vi "bah.vi"() -> ()   [LabVIEW 2013]
panel:
  in  "OK Button 2":bool
  in  "Один раз(T)/50 раз (F)":bool
  in  "МОЩА":dbl=50.0
  in  "БАХНУТЬ":bool
  in  "OK Button":bool
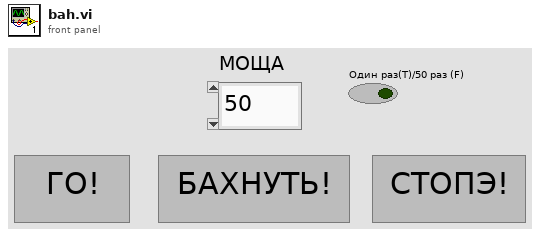
[diagram p1: front panel]
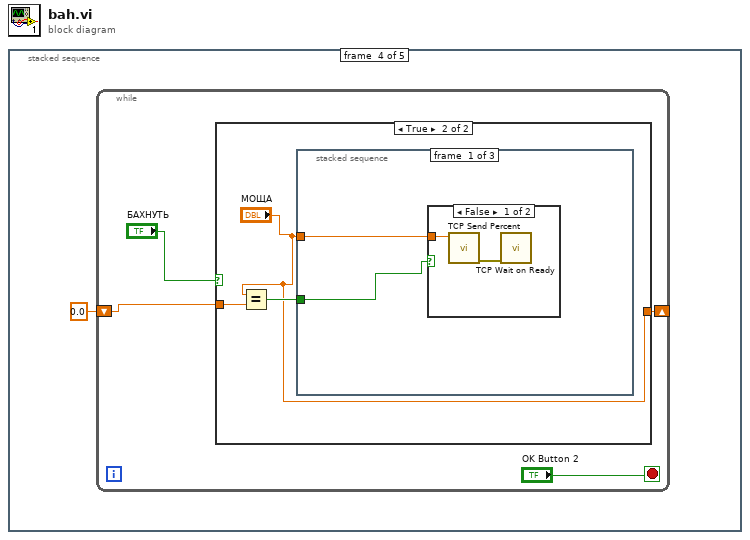
[diagram p0: block diagram]
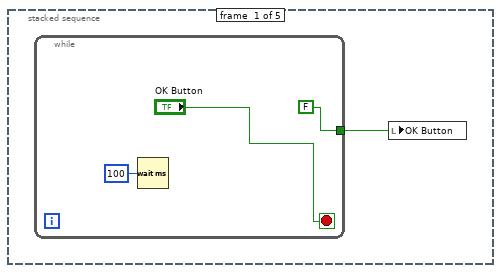
[diagram p2: hidden frame]
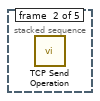
[diagram p3: hidden frame]
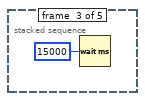
[diagram p4: hidden frame]
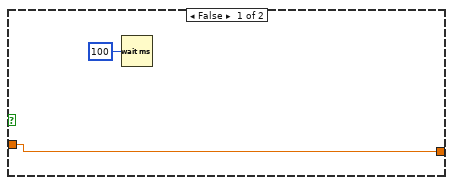
[diagram p5: hidden frame]
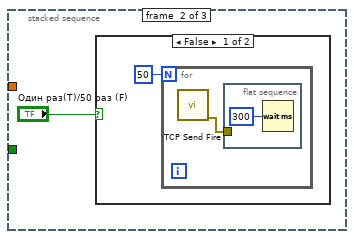
[diagram p7: hidden frame]
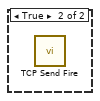
[diagram p8: hidden frame]
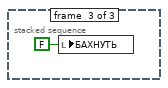
[diagram p9: hidden frame]
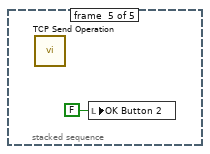
[diagram p10: hidden frame]
diagram:
  n1 = stacked-sequence {
    frame #0 {
      n2 = while {
        tunnel: [FALSE] -> w1
        stop <- "OK Button" stop-if-true
        n3 = Wait (ms)(milliseconds to wait=u32 100) -> ()  [unwired: 1 out]
      }
      n4 = local write "OK Button"(w1) -> ()
    }
    frame #1 {
      n5 = call "TCP Send Operation.vi"() -> ()  [unwired: 11 in, 1 out]
    }
    frame #2 {
      n6 = Wait (ms)(milliseconds to wait=u32 15000) -> ()  [unwired: 1 out]
    }
    frame #3 {
      n7 = while {
        shift-right: [w7] -> _
        shift-left: 0.0 ("МОЩА") -> [w8]
        stop <- "OK Button 2" stop-if-true
        n8 = case shown="True" "БАХНУТЬ" {
          tunnel: w8 -> [w11 w15]
          tunnel: [w11 "МОЩА"] -> w7
          frame False {
            n9 = Wait (ms)(milliseconds to wait=u32 100) -> ()  [unwired: 1 out]
          }
          frame True {
            n10 = Equal?(x="МОЩА", y=w15) -> (x = y?=w14:bool)
            n11 = stacked-sequence {
              tunnel: w14 -> [w17 _ _]
              tunnel: "МОЩА" -> [w16 _ _]
              frame #0 {
                n12 = case shown="False" w17 {
                  tunnel: w16 -> [w18 _]
                  frame False {
                    n13 = call "TCP Send Percent.vi"("Percent"=w18) -> ("error out"=w19:errorcluster)  [unwired: 10 in]
                    n14 = call "TCP Wait on Ready.vi"("error in"=w19) -> ()  [unwired: 9 in, 1 out]
                  }
                  frame True {
                  }
                }
              }
              frame #1 {
                n15 = case shown="False" "Один раз(T)/50 раз (F)" {
                  frame False {
                    n16 = for {
                      N: 50 -> [_]
                      n17 = call "TCP Send Fire.vi"() -> ("error out"=w22:errorcluster)  [unwired: 11 in]
                      n18 = flat-sequence {
                        tunnel: w22 -> [_]
                        frame #0 {
                          n19 = Wait (ms)(milliseconds to wait=u32 300) -> ()  [unwired: 1 out]
                        }
                      }
                    }
                  }
                  frame True {
                    n20 = call "TCP Send Fire.vi"() -> ()  [unwired: 11 in, 1 out]
                  }
                }
              }
              frame #2 {
                n21 = local write "БАХНУТЬ"(FALSE ("БАХНУТЬ")) -> ()
              }
            }
          }
        }
      }
    }
    frame #4 {
      n22 = call "TCP Send Operation.vi"() -> ()  [unwired: 11 in, 1 out]
      n23 = local write "OK Button 2"(FALSE ("OK Button 2")) -> ()
    }
  }
